vi "ChangeColor.vi"(8 "error in (no error)":errorcluster, 11 "MCListbox Refnum":refnum<vi>) -> (0 "error out":errorcluster)   [LabVIEW 2011]
uses:
  <vilib>/Utility/miscctls.llb/LVRowAndColumnTypeDef.ctl
panel:
  in  "偶数字体":u32(colorbox)
  in  "偶数背景":u32(colorbox)
  in  "奇数背景":u32(colorbox)
  in  "奇数字体":u32(colorbox)
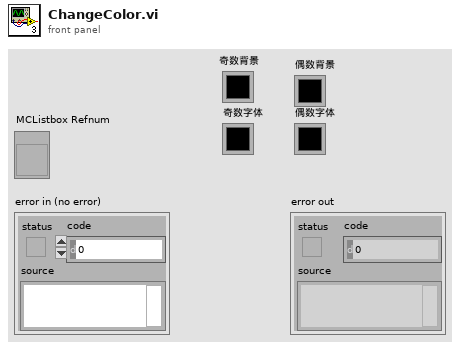
[diagram p1: front panel]
types:
  T1 = typedef "LVRowAndColumnTypeDef.ctl" = cluster{"Row":i32, "Column":i32}
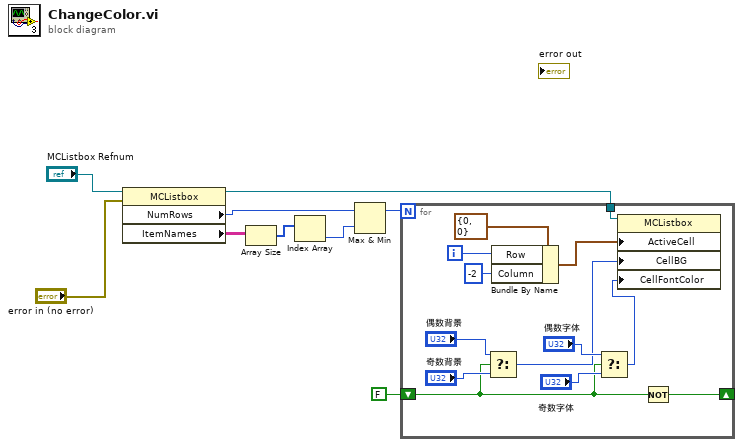
[diagram p0: block diagram]
diagram:
  n1 = property class="MCListbox"(reference="MCListbox Refnum", error in="error in (no error)") -> (reference out=w2:refnum<vi>, "NumRows"=w4:u32, "ItemNames"=w7:string[][])  [unwired: 1 out]
  n2 = Array Size(array=w7) -> (size(s)=w6:i32[])
  n3 = Index Array(array=w6) -> (element=w5:i32)  [unwired: 1 in]
  n4 = Max & Min(x=w4, y=w5) -> (max(x,y)=w3:u32)  [unwired: 1 out]
  n5 = for {
    N: w3 -> [_]
    tunnel: w2 -> [w17]
    shift-right: [w10] -> _
    shift-left: FALSE -> [w18]
    i -> [w14]
    n6 = Select(t="偶数背景", s=w18, f="奇数背景") -> (s? t:f=w11:u32)
    n7 = Bundle By Name(cluster=T1 {"Row"=0, "Column"=0} ("Active Cell:Active Cell"), "Row"=w14, "Column"=-2) -> (w15:T1)
    n8 = Select(t="偶数字体", s=w18, f="奇数字体") -> (s? t:f=w12:u32)
    n9 = property class="MCListbox"(reference=w17, "ActiveCell"=w15, "CellBG"=w11, "CellFontColor"=w12) -> ()  [unwired: 1 in, 2 out]
    n10 = Not(x=w18) -> (.not. x?=w10:bool)
  }
